vi "chamber_out.vi"   [LabVIEW 2013]
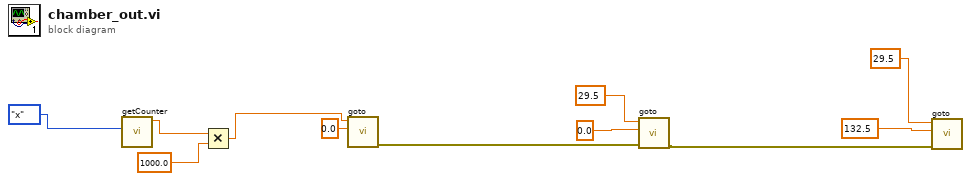
[diagram p0: block diagram]
diagram:
  n1 = call "getCounter.vi"("channel"=enum16{"x", "y"}."x" ("axie")) -> ("result"=w3:dbl)  [unwired: 9 in, 1 out]
  n2 = Multiply(x=w3, y=1000.0) -> (x*y=w1:dbl)
  n3 = call "goto.vi"("Y(mm)"=0.0, "X(mm)"=w1) -> ("错误输出"=w8:errorcluster)  [unwired: 9 in]
  n4 = call "goto.vi"("错误输入（无错误）"=w8, "Y(mm)"=0.0, "X(mm)"=29.5) -> ("错误输出"=w6:errorcluster)  [unwired: 8 in]
  n5 = call "goto.vi"("错误输入（无错误）"=w6, "Y(mm)"=132.5, "X(mm)"=29.5) -> ()  [unwired: 8 in, 1 out]
